vi "Create Signal Properties - Dual Tone.vi"(8 "error in (no error)":errorcluster, 10 "dual tone properties":T1, 11 "AudioGeneration in":refnum<class "AudioGeneration.lvclass">) -> (0 "error out":errorcluster, 2 "signal settings":T3, 3 "AudioGeneration out":refnum<class "AudioGeneration.lvclass">)   [LabVIEW 2021, in "AudioGeneration.lvclass"]
uses:
  AudioGeneration.lvclass
  controls/signal settings.ctl
  controls/signal type.ctl
  shared/controls/digital output level units.ctl
  AudioGeneration.lvclass/AudioGeneration.ctl
  controls/AudioGenTypeDefs.lvlib
  shared/controls/audio controls.lvlib
  controls/dual tone types.ctl
  controls/dual tone properties.ctl
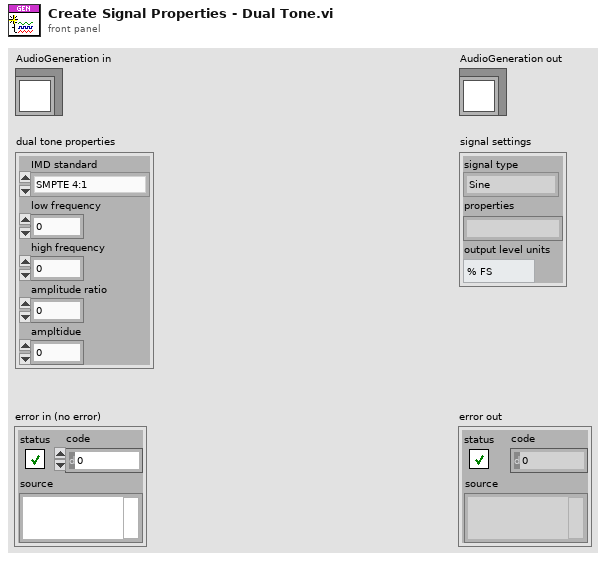
[diagram p1: front panel]
types:
  T1 = typedef "AudioGenTypeDefs.lvlib/dual tone properties.ctl" = cluster{"IMD standard":T2, "low frequency":dbl, "high frequency":dbl, "amplitude ratio":dbl, "ampltidue":dbl}
  T2 = typedef "AudioGenTypeDefs.lvlib/dual tone types.ctl" = enum32{"SMPTE 4:1", "DIN", "CCIF 11k-12k", "CCIF 19k-20k", "Custom"}
  T3 = typedef "AudioGenTypeDefs.lvlib/signal settings.ctl" = cluster{"signal type":T4, "properties":string, "output level units":T5}
  T4 = typedef "AudioGenTypeDefs.lvlib/signal type.ctl" = enum16{"Sine", "Dual Tone"}
  T5 = typedef "audio controls.lvlib/digital output level units.ctl" = enum32{"% FS", "dBFS", "V"}
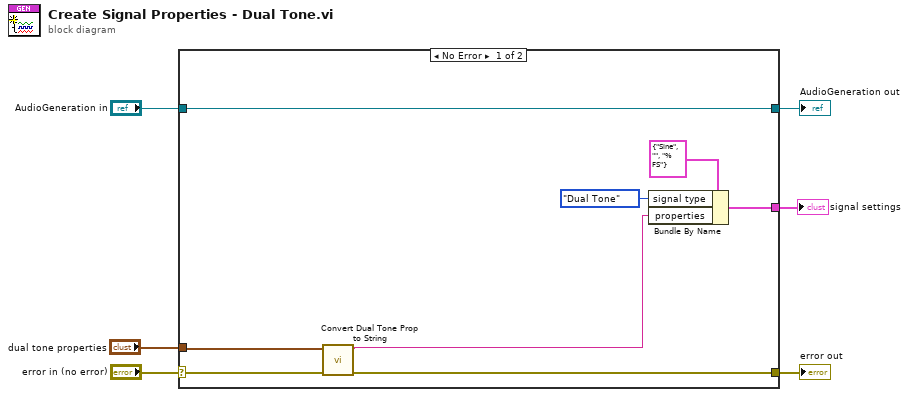
[diagram p0: block diagram]
diagram:
  n1 = case shown="No Error" "error in (no error)" {
    selector: "error in (no error)" -> [w10 w16]
    tunnel: [w9 w16] -> w5
    tunnel: [w14 w15] -> w3
    tunnel: "AudioGeneration in" -> [w14 w15]
    tunnel: [w12 _] -> w2
    tunnel: "dual tone properties" -> [w7 _]
    frame No Error {
      n2 = call "Convert Dual Tone Prop to String.vi"("error in (no error)"=w10, "dual tone properties"=w7) -> ("error out"=w9:errorcluster, "dual tone properties"=w8:string)  [unwired: 8 in]
      n3 = Bundle By Name(cluster=T3 {"signal type"=enum."Sine", "properties"="", "output level units"=enum."% FS"} ("signal settings"), "signal type"=signal_type."Dual Tone", "properties"=w8) -> (w12:T3)
    }
    frame Error {
    }
  }
  "error out" <- w5
  "AudioGeneration out" <- w3
  "signal settings" <- w2
